vi "Temperature Warnings.vi"(11 "wejscie":T1={"Current Temperature"=0.0, "Max Temperature"=0.0, "Min Temperature"=0.0, "Warning?"=FALSE, "Warning Text"="No Warning", "Error In"={"status"=FALSE, "code"=0, "source"=""}, "Error Out"={"status"=FALSE, "code"=0, "source"=""}}) -> ()   [LabVIEW 2015]
doc: "This VI is used to determine the string to output to the weather station based on the current temperature and limit settings.\n\nInputs: Current Temperature (DBL), Minimum Temperature (DBL), and Maximum Temperature (DBL).\nOutputs: Warning Text (string) and Warning? (Boolean)."
panel:
  out "wyjscie":T1={"Current Temperature"=0.0, "Max Temperature"=0.0, "Min Temperature"=0.0, "Warning?"=FALSE, "Warning Text"="No Warning", "Error In"={"status"=FALSE, "code"=0, "source"=""}, "Error Out"={"status"=FALSE, "code"=0, "source"=""}}
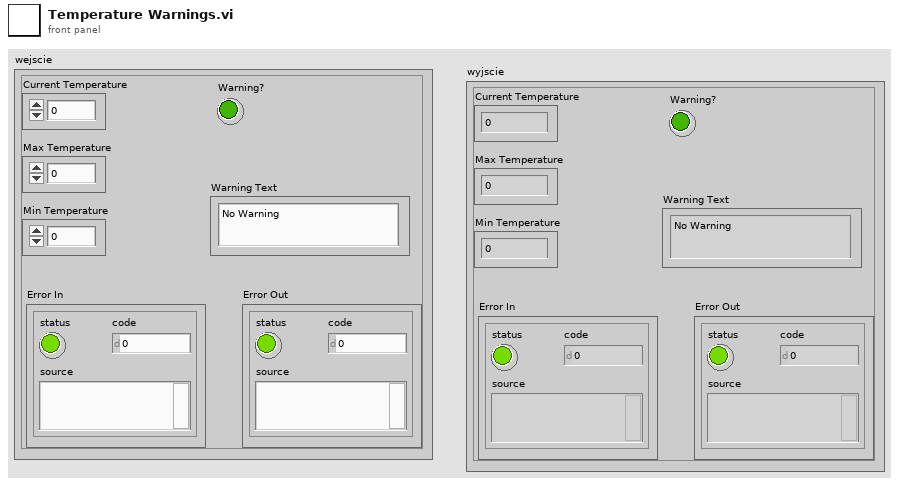
[diagram p1: front panel]
types:
  T1 = cluster{"Current Temperature":dbl, "Max Temperature":dbl, "Min Temperature":dbl, "Warning?":bool, "Warning Text":string, "Error In":errorcluster, "Error Out":errorcluster}
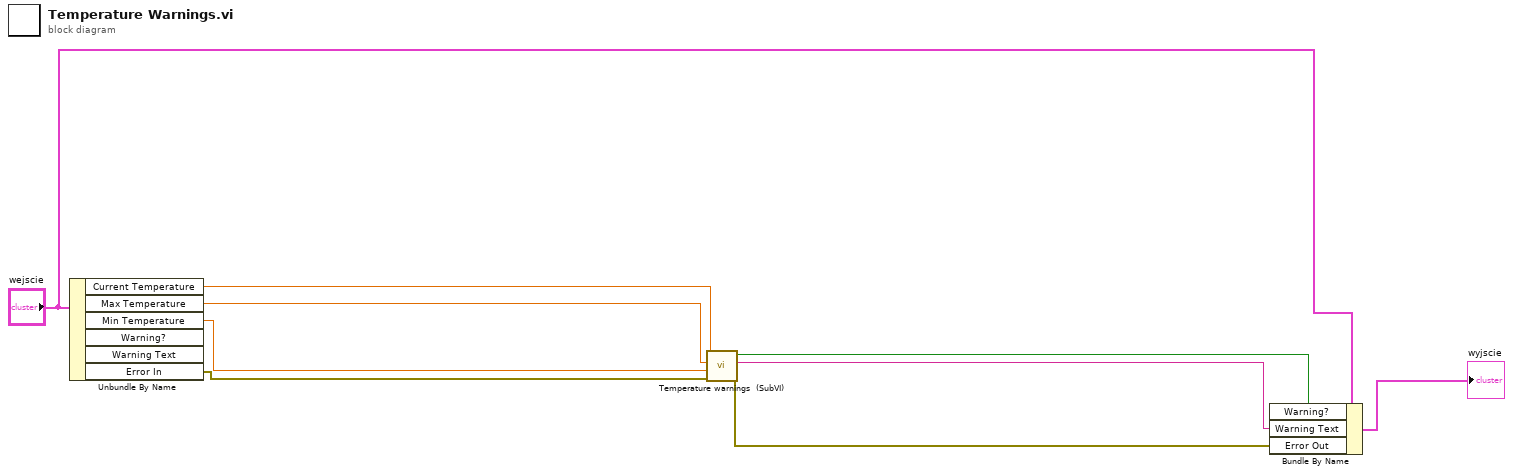
[diagram p0: block diagram]
diagram:
  n1 = Unbundle By Name("wejscie") -> ("Current Temperature"=w8:dbl, "Max Temperature"=w7:dbl, "Min Temperature"=w6:dbl, "Error In"=w9:errorcluster)  [unwired: 2 out]
  n2 = call "Temperature warnings  (SubVI).vi"("error in (no error)"=w9, "Min Temperature"=w6, "Max Temperature"=w7, "Current Temperature"=w8) -> ("error out"=w3:errorcluster, "f"=w1:string, "Boolean"=w2:bool)  [unwired: 5 in]
  n3 = Bundle By Name(cluster="wejscie", "Warning?"=w2, "Warning Text"=w1, "Error Out"=w3) -> (→"wyjscie":T1)
